vi "GetHWInfo.vi"(8 "error in":errorcluster caption="error in (no error)") -> (0 "error out":errorcluster, 3 "Refs Out":variant)   [LabVIEW 2011]
uses:
  Controls/ModuleCluster.ctl
  <vilib>/nisyscfg/Initialize (Control).vi
  <vilib>/nisyscfg/Find Hardware.vi
  <vilib>/nisyscfg/nisyscfg.lvlib
  Program Files/National Instruments/LabVIEW 2011/resource/objmgr/nisysapi.rc
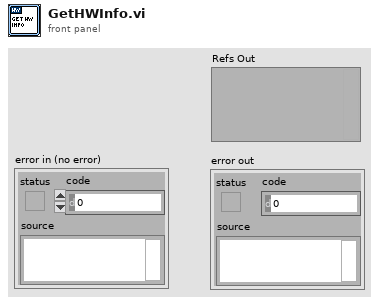
[diagram p1: front panel]
types:
  T1 = typedef "ModuleCluster.ctl" = cluster{"Device Ref":refnum<k20>, "ProdName":string, "ConnLink":string, "Alias":string}
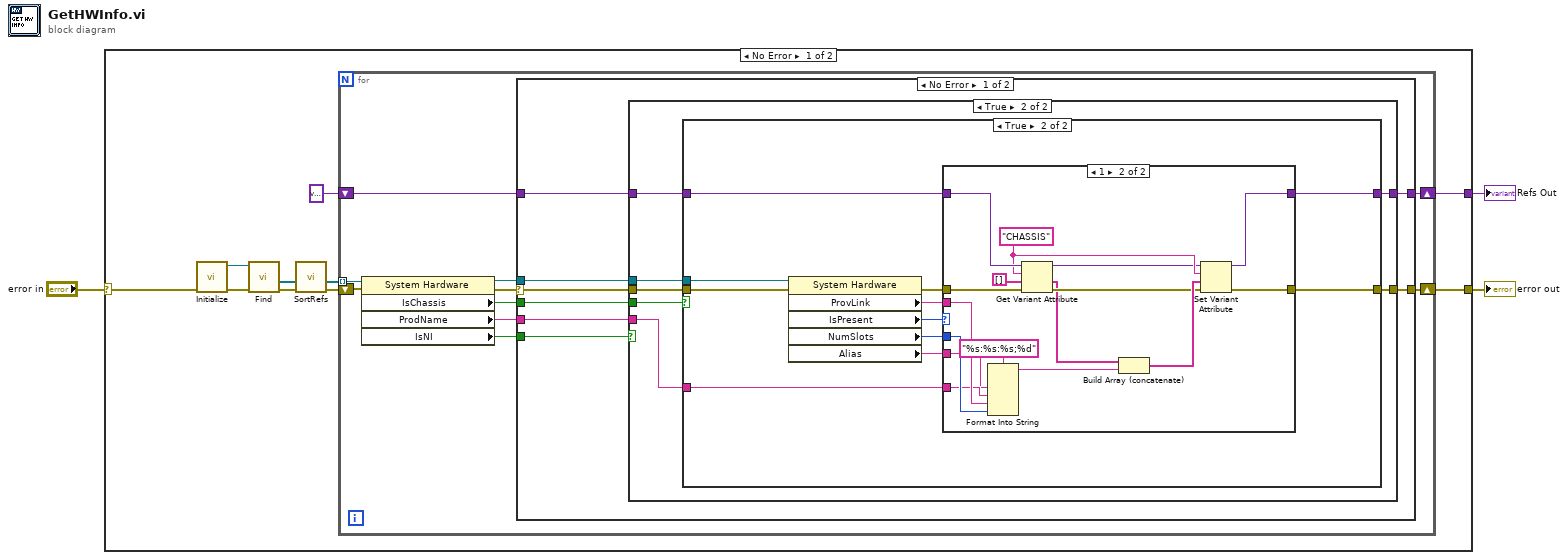
[diagram p0: block diagram]
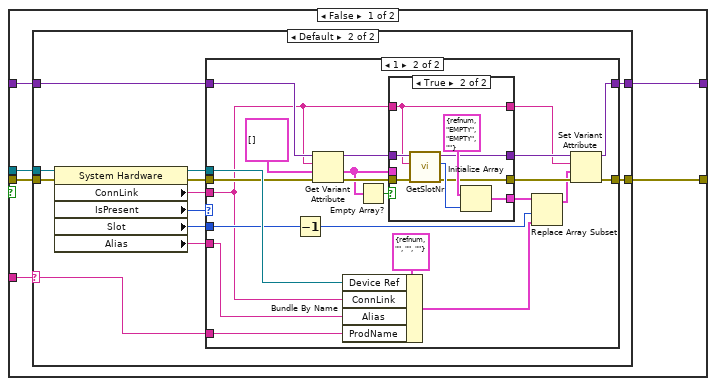
[diagram p3: hidden frame]
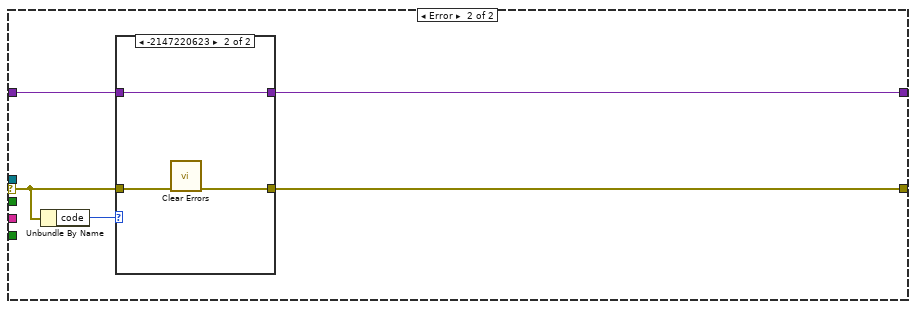
[diagram p8: hidden frame]
diagram:
  n1 = case shown="No Error" "error in" {
    selector: "error in" -> [w9 w135]
    tunnel: [w11 _] -> w3
    tunnel: [w10 w135] -> w2
    frame No Error {
      n2 = call-poly <vilib>:"Initialize.vi"("error in (no error)"=w9) -> ("error out"=w12:errorcluster, "session out"=w8:refnum<k21>)  [unwired: 8 in, 1 out]
      n3 = call-poly <vilib>:"Find.vi"("error in (no error)"=w12, "session in"=w8) -> ("error out"=w5:errorcluster, "resources out"=w7:refnum<k20>[])  [unwired: 6 in, 2 out]
      n4 = call "SortRefs.vi"("error in"=w5, "Refs In"=w7) -> ("error out"=w4:errorcluster, "Refs Out"=w6:refnum<k20>[])  [unwired: 8 in]
      n5 = for {
        tunnel: w6 -> [w15] mode=indexing
        shift-right: [w19] -> w11
        shift-left: variant ("variant") -> [w21]
        shift-right: [w16] -> w10
        shift-left: w4 -> [w17]
        n6 = property class="System Hardware"(reference=w15, error in=w17) -> (reference out=w18:refnum<k20>, error out=w14:errorcluster, "IsChassis"=w22:bool, "ProdName"=w20:string, "IsNI"=w23:bool)
        n7 = case shown="No Error" w14 {
          selector: w14 -> [w24 w129]
          tunnel: w23 -> [w31 _]
          tunnel: w22 -> [w30 _]
          tunnel: w21 -> [w29 w127]
          tunnel: w20 -> [w28 _]
          tunnel: [w27 w126] -> w19
          tunnel: w18 -> [w26 _]
          tunnel: [w25 w128] -> w16
          frame No Error {
            n8 = case shown="True" w31 {
              tunnel: w30 -> [_ w40]
              tunnel: w29 -> [w33 w39]
              tunnel: w28 -> [_ w38]
              tunnel: [w33 w37] -> w27
              tunnel: w26 -> [_ w36]
              tunnel: w24 -> [w32 w35]
              tunnel: [w32 w34] -> w25
              frame False {
              }
              frame True {
                n9 = case shown="True" w40 {
                  tunnel: w39 -> [w45 w107]
                  tunnel: w38 -> [w41 w102]
                  tunnel: [w46 w106] -> w37
                  tunnel: w36 -> [w42 w104]
                  tunnel: w35 -> [w43 w103]
                  tunnel: [w44 w105] -> w34
                  frame False {
                    n10 = case shown="Default" w41 {
                      selector: w41 -> [_ w50]
                      tunnel: [w47 w60] -> w46
                      tunnel: w45 -> [w47 w59]
                      tunnel: [w48 w58] -> w44
                      tunnel: w43 -> [w48 w57]
                      tunnel: w42 -> [_ w55]
                      frame "NI cDAQ-9188" {
                        # "No Ethernet devices yet implemented"
                      }
                      frame Default {
                        n11 = property class="System Hardware"(reference=w55, error in=w57) -> (reference out=w54:refnum<k20>, error out=w56:errorcluster, "ConnLink"=w53:string, "IsPresent"=w52:i32, "Slot"=w51:i32, "Alias"=w49:string)
                        n12 = case shown="1" w52 {
                          tunnel: w50 -> [_ w64]
                          tunnel: [w62 w83] -> w60
                          tunnel: w59 -> [w62 w78]
                          tunnel: [w61 w81] -> w58
                          tunnel: w56 -> [w61 w79]
                          tunnel: w54 -> [_ w80]
                          tunnel: w53 -> [_ w66]
                          tunnel: w51 -> [_ w68]
                          tunnel: w49 -> [_ w63]
                          frame Default {
                          }
                          frame 1 {
                            n13 = Decrement(x=w68) -> (x-1=w65:i32)
                            n14 = Get Variant Attribute(Variant=w78, name=w66, default value (empty Variant)=T1[] [] ("appended array"), error in=w79) -> (duplicate Variant=w75:variant, value=w73:T1[], error out=w77:errorcluster)  [unwired: 1 out]
                            n15 = Bundle By Name(cluster=T1 {"Device Ref"=refnum, "ProdName"="", "ConnLink"="", "Alias"=""} ("module cluster"), "Device Ref"=w80, "ConnLink"=w66, "Alias"=w63, "ProdName"=w64) -> (w67:T1)
                            n16 = Empty Array?(array=w73) -> (empty?=w76:bool)
                            n17 = case shown="True" w76 {
                              tunnel: w77 -> [w86 w96]
                              tunnel: w75 -> [w88 w95]
                              tunnel: [w88 w91] -> w74
                              tunnel: w73 -> [w87 _]
                              tunnel: [w87 w92] -> w70
                              tunnel: [w86 w90] -> w72
                              tunnel: w66 -> [w85 w89]
                              tunnel: [w85 w89] -> w71
                              frame False {
                              }
                              frame True {
                                n18 = call "GetSlotNr.vi"("Error In"=w96, "Variable In"=w89, "Variant In"=w95) -> ("Error Out"=w90:errorcluster, "Nr of Slots Out"=w93:i32, "Variant Out"=w91:variant)  [unwired: 6 in]
                                n19 = Initialize Array(T1 {"Device Ref"=refnum, "ProdName"="EMPTY", "ConnLink"="EMPTY", "Alias"=""} ("module cluster"), w93) -> (w92:T1[])
                              }
                            }
                            n20 = Replace Array Subset(array=w70, new element=w67, index=w65) -> (w69:T1[])
                            n21 = Set Variant Attribute(Variant=w74, name=w71, value=w69, error in=w72) -> (Variant out=w83:variant, error out=w81:errorcluster)  [unwired: 1 out]
                          }
                        }
                      }
                    }
                  }
                  frame True {
                    n22 = property class="System Hardware"(reference=w104, error in=w103) -> (error out=w100:errorcluster, "ProvLink"=w101:string, "IsPresent"=w99:i32, "NumSlots"=w98:i32, "Alias"=w97:string)  [unwired: 1 out]
                    n23 = case shown="1" w99 {
                      tunnel: w107 -> [w109 w125]
                      tunnel: [w109 w120] -> w106
                      tunnel: [w108 w118] -> w105
                      tunnel: w101 -> [_ w112]
                      tunnel: w102 -> [_ w111]
                      tunnel: w100 -> [w108 w115]
                      tunnel: w98 -> [_ w113]
                      tunnel: w97 -> [_ w110]
                      frame Default {
                      }
                      frame 1 {
                        w123 = "CHASSIS" ("name")
                        n24 = Format Into String(format string="%s:%s:%s;%d", w110, w111, w112, w113) -> (resulting string=w116:string)  [unwired: 2 in, 1 out]
                        n25 = Get Variant Attribute(Variant=w125, name=w123, default value (empty Variant)=string[] [], error in=w115) -> (duplicate Variant=w122:variant, value=w114:string[], error out=w119:errorcluster)  [unwired: 1 out]
                        n26 = Build Array (concatenate)(w114, w116) -> (w121:string[])
                        n27 = Set Variant Attribute(Variant=w122, name=w123, value=w121, error in=w119) -> (Variant out=w120:variant, error out=w118:errorcluster)  [unwired: 1 out]
                      }
                    }
                  }
                }
              }
            }
          }
          frame Error {
            n28 = Unbundle By Name(w129) -> ("code"=w130:i32)
            n29 = case shown="-2147220623" w130 {
              tunnel: w129 -> [w131 w134]
              tunnel: [w131 w133] -> w128
              tunnel: w127 -> [_ w132]
              tunnel: [_ w132] -> w126
              frame Default {
              }
              frame -2147220623 {
                n30 = call <vilib>:"Clear Errors.vi"("error in (no error)"=w134) -> ("error out"=w133:errorcluster)  [unwired: 6 in]
              }
            }
          }
        }
      }
    }
    frame Error {
    }
  }
  "Refs Out" <- w3
  "error out" <- w2
